vi "Go Straight.vi"(4 "Right Motor In":dbl=-0.0, 5 "Left Motor In":dbl=-0.0) -> (1 "Right Motor Out":dbl=-0.0, 2 "Left Motor Out":dbl=-0.0)   [LabVIEW 2012]
uses:
  Robot Global Data.vi
  <vilib>/addons/control/pid/pid.llb/PID (DBL).vi
  <vilib>/addons/control/pid/NI_PID_pid.lvlib
panel:
  in  "StraightPID gains":T1={"proportional gain (Kc)"=2.0, "integral time (Ti, min)"=0.0, "derivative time (Td, min)"=0.0} {"derivative time (Td, min)" format="%.3f"; "integral time (Ti, min)" format="%.3f"; "proportional gain (Kc)" format="%.3f"}
  out "Header":dbl=210.23117651851842
  # "The gain and PID gains are redundant"
  # "300*.025 = 7.5"
  # "2.0"
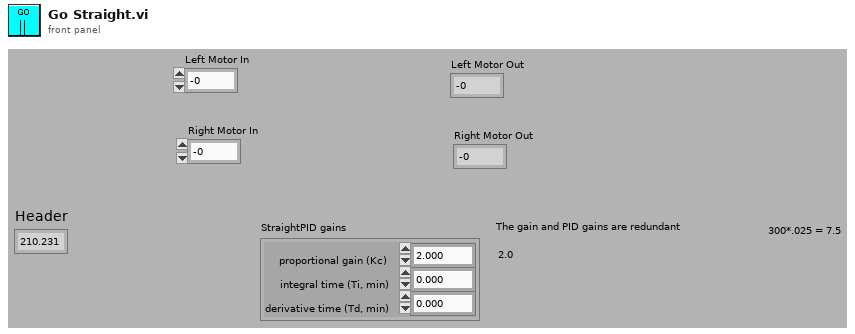
[diagram p1: front panel]
types:
  T1 = cluster{"proportional gain (Kc)":dbl, "integral time (Ti, min)":dbl, "derivative time (Td, min)":dbl}
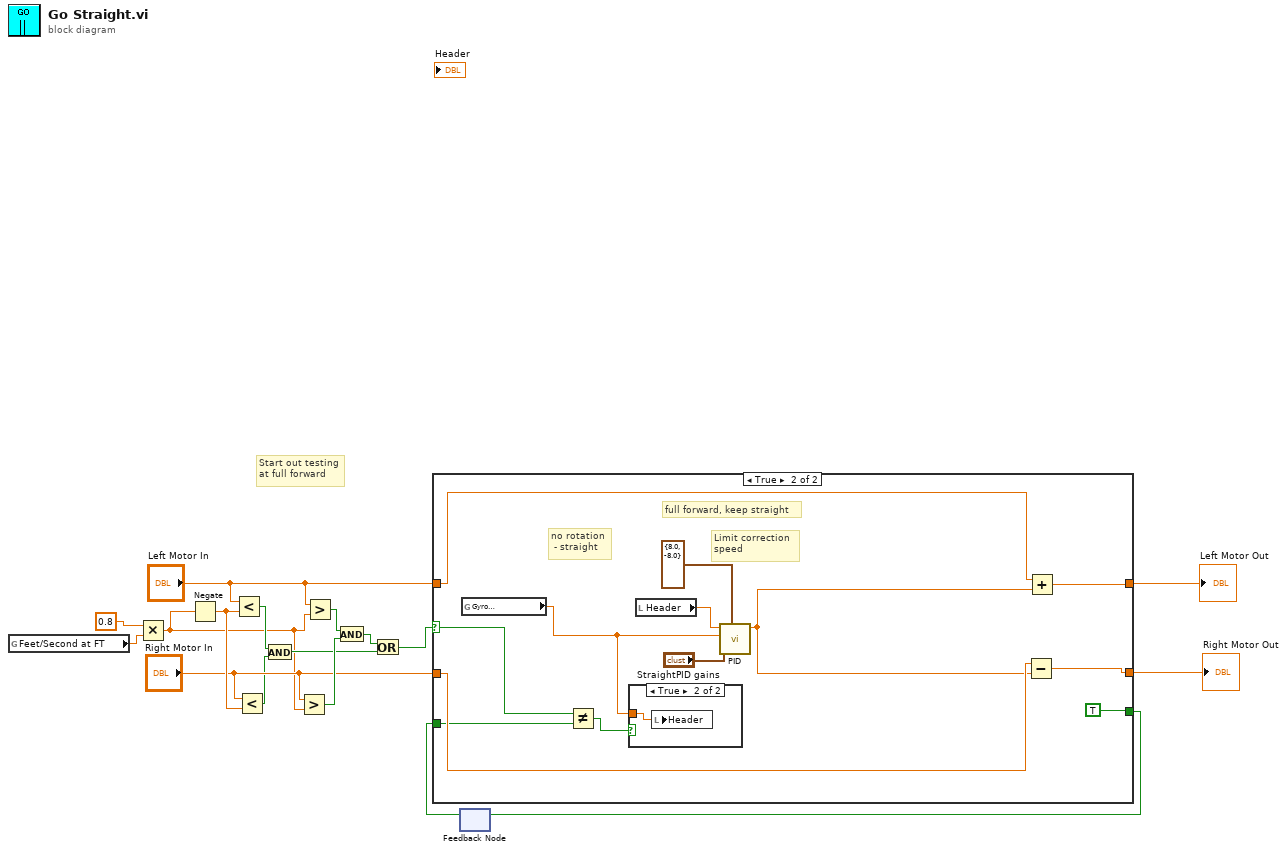
[diagram p0: block diagram]
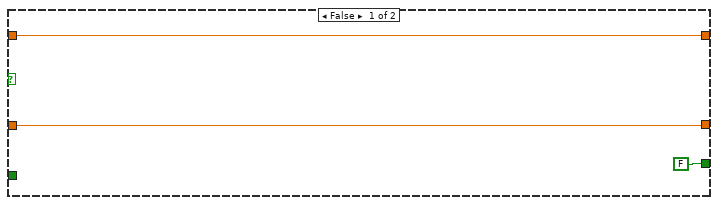
[diagram p2: hidden frame]
diagram:
  # "Start out testing\nat full forward"
  n1 = global read "Robot Global Data.vi" "Feet/Second at FT"() -> (w2:dbl)
  n2 = Multiply(x=0.8 ("Speed to Go straight at"), y=w2) -> (x*y=w1:dbl)
  n3 = Negate(x=w1) -> (-x=w10:dbl)
  n4 = Less?(x="Left Motor In", y=w10) -> (x < y?=w8:bool)
  n5 = Less?(x="Right Motor In", y=w10) -> (x < y?=w7:bool)
  n6 = And(x=w8, y=w7) -> (x .and. y?=w5:bool)
  n7 = Greater?(x="Right Motor In", y=w1) -> (0:w14:bool)
  n8 = Greater?(x="Left Motor In", y=w1) -> (0:w15:bool)
  n9 = And(x=w15, y=w14) -> (x .and. y?=w6:bool)
  n10 = Or(x=w6, y=w5) -> (x .or. y?=w4:bool)
  n11 = feedback #1() -> (w13:bool)  [unwired: 1 out]
  n12 = case shown="True" w4 {
    selector: w4 -> [_ w27]
    tunnel: [w19 w32] -> w17
    tunnel: [w20 w31] -> w16
    tunnel: "Left Motor In" -> [w20 w30]
    tunnel: "Right Motor In" -> [w19 w29]
    tunnel: [FALSE TRUE] -> w12
    tunnel: w13 -> [_ w26]
    frame False {
    }
    frame True {
      # "Limit correction\nspeed"
      # "no rotation\n - straight"
      # "full forward, keep straight"
      n13 = global read "Robot Global Data.vi" "Gyro\nAngle"() -> (w28:dbl)
      n14 = Not Equal?(x=w27, y=w26) -> (x != y?=w25:bool)
      n15 = case shown="True" w25 {
        tunnel: w28 -> [_ w34]
        frame False {
        }
        frame True {
          n16 = local write "Header"(w34) -> ()
        }
      }
      n17 = local read "Header"() -> (w23:dbl)
      n18 = call-poly <vilib>:"PID.vi"("output range"=cluster{"output high":dbl, "output low":dbl} {"output high"=8.0, "output low"=-8.0}, "PID gains"="StraightPID gains", "process variable"=w28, "setpoint"=w23) -> ("output"=w21:dbl)  [unwired: 2 in, 5 out]
      n19 = Subtract(x=w29, y=w21) -> (x-y=w32:dbl)
      n20 = Add(x=w30, y=w21) -> (x+y=w31:dbl)
    }
  }
  "Left Motor Out" <- w16
  "Right Motor Out" <- w17
  n21 = feedback-in #1(w12) -> ()
